vi "set_selected_ROI.vi"(8 "error in (no error)":errorcluster, 10 "RoiGeneric.lvclass":refnum<class "RoiGeneric.lvclass">, 11 "RoiCollection in":refnum<class "RoiCollection.lvclass">) -> (0 "error out":errorcluster, 3 "RoiCollection out":refnum<class "RoiCollection.lvclass">)   [LabVIEW 2010, in "RoiCollection.lvclass"]
uses:
  RoiCollection.lvclass
  RoiGeneric/RoiGeneric.lvclass
  RoiCollection.lvclass/RoiCollection.ctl
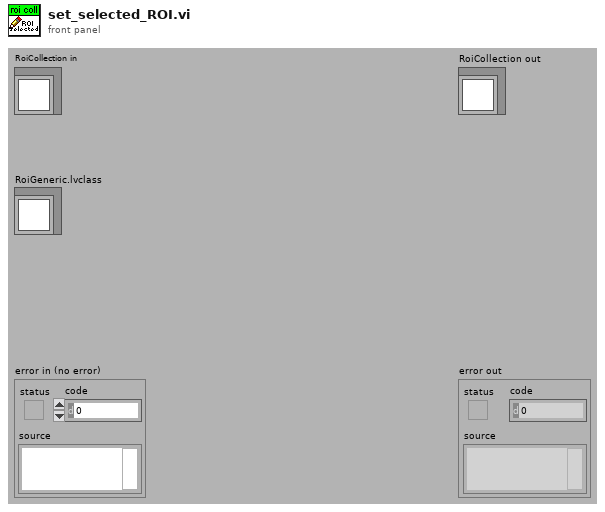
[diagram p1: front panel]
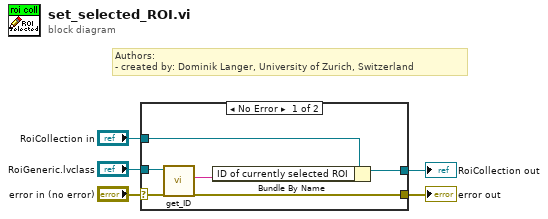
[diagram p0: block diagram]
diagram:
  # "Authors: \n- created by: Dominik Langer, University of Zurich, Switzerland"
  n1 = case shown="No Error" "error in (no error)" {
    selector: "error in (no error)" -> [w11 w13]
    tunnel: [w10 w13] -> w4
    tunnel: [w6 w12] -> w2
    tunnel: "RoiCollection in" -> [w7 w12]
    tunnel: "RoiGeneric.lvclass" -> [w9 _]
    frame No Error {
      n2 = call-dynamic "get_ID.vi"("error in (no error)"=w11, "RoiGeneric in"=w9) -> ("error out"=w10:errorcluster, "ID"=w8:string)  [unwired: 7 in, 1 out]
      n3 = Bundle By Name(cluster=w7, "ID of currently selected ROI"=w8) -> (w6:refnum<class "RoiCollection.lvclass">)
    }
    frame Error {
    }
  }
  "error out" <- w4
  "RoiCollection out" <- w2
